vi "getAdditionalDataFromXMLNative.vi"(8 "error in (no error)":errorcluster, 10 "eventXML":refnum<k20>, 11 "PlayFile in":refnum<class "PlayFile.lvclass">) -> (0 "error out":errorcluster, 2 "eventXML out":refnum<k20>, 3 "PlayFile out":refnum<class "PlayFile.lvclass">)   [LabVIEW 2011, in "Tools.lvlib" / "Scripting.lvlib" / "PlayFile.lvclass"]
uses:
  PlayFile.lvclass
  PlayFile.lvclass/PlayFile.ctl
  <vilib>/xml/Close Reference(Node).vi
  <vilib>/xml/NI_XML.lvlib
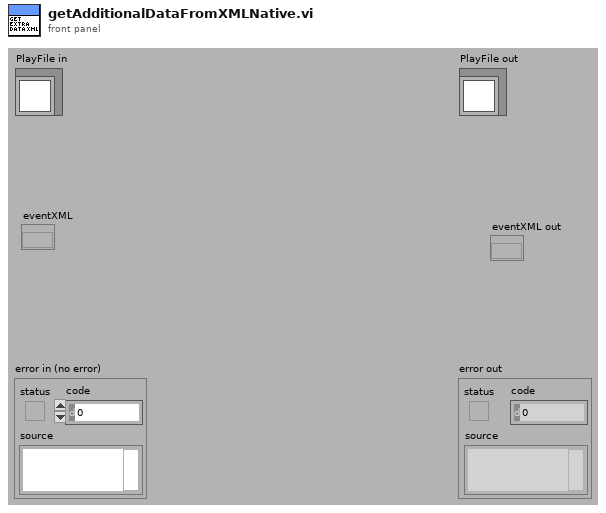
[diagram p1: front panel]
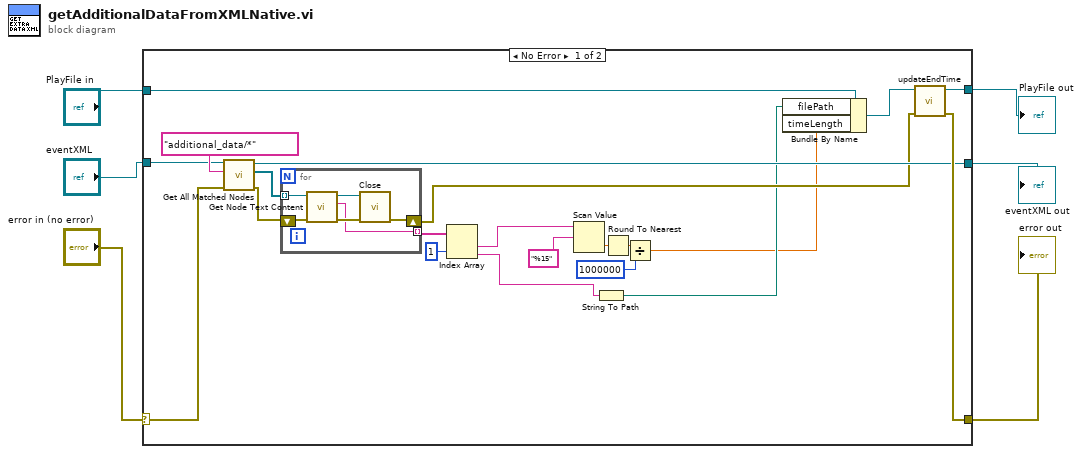
[diagram p0: block diagram]
diagram:
  n1 = case shown="No Error" "error in (no error)" {
    selector: "error in (no error)" -> [w14 w34]
    tunnel: [w21 w34] -> w3
    tunnel: "PlayFile in" -> [w25 w35]
    tunnel: [w22 w35] -> w2
    tunnel: "eventXML" -> [w15 _]
    tunnel: [w13 _] -> w1
    frame No Error {
      n2 = call <vilib>:"Get All Matched Nodes.vi"("error in (no error)"=w14, "XPath expression"="additional_data/*", "node in"=w15) -> ("error out"=w20:errorcluster, "node result array"=w18:refnum<k20>[], "node out"=w13:refnum<k20>)  [unwired: 6 in]
      n3 = for {
        tunnel: w18 -> [w30] mode=indexing
        tunnel: [w29] -> w17 mode=indexing
        shift-right: [w28] -> w11
        shift-left: w20 -> [w31]
        n4 = call <vilib>:"Get Node Text Content.vi"("error in (no error)"=w31, "node in"=w30) -> ("error out"=w32:errorcluster, "node text"=w29:string, "node out"=w33:refnum<k20>)  [unwired: 7 in]
        n5 = call-poly <vilib>:"Close.vi"("error in (no error)"=w32, "node"=w33) -> ("error out"=w28:errorcluster)  [unwired: 7 in]
      }
      n6 = Index Array(array=w17, index #2=1 ("index")) -> (element #1=w12:string, element #2=w9:string)  [unwired: 1 in]
      n7 = Scan Value(string=w12, format string="%15") -> (value=w27:dbl)  [unwired: 1 in, 1 out]
      n8 = String To Path(string=w9) -> (path=w8:path)
      n9 = Round To Nearest(number=w27) -> (nearest integer value=w10:dbl)
      n10 = Divide(x=w10, y=1000000) -> (x/y=w7:dbl)
      n11 = Bundle By Name(cluster=w25, "filePath"=w8, "timeLength"=w7) -> (w23:refnum<class "PlayFile.lvclass">)
      n12 = call-dynamic "updateEndTime.vi"("error in (no error)"=w11, "ScriptEvent in"=w23) -> ("error out"=w21:errorcluster, "ScriptEvent out"=w22:refnum<class "PlayFile.lvclass">)  [unwired: 8 in]
    }
    frame Error {
    }
  }
  "error out" <- w3
  "PlayFile out" <- w2
  "eventXML out" <- w1
